vi "VFD.vi"   [LabVIEW 2018]
uses:
  CRC16/CRC16Settings.ctl
types:
  T1 = typedef "CRC16Settings.ctl" = cluster{"DataFIFO":refnum<k21>, "CalculateFIFO":refnum<k21>, "CRCFIFO":refnum<k21>}
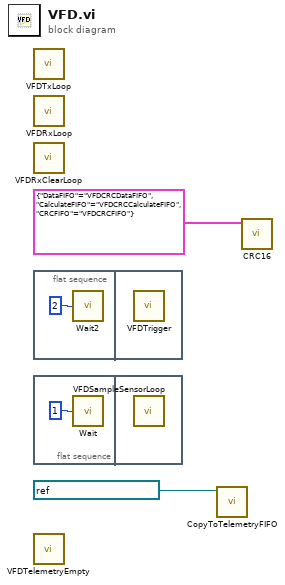
[diagram p0: block diagram]
diagram:
  n1 = call "VFDTxLoop.vi"() -> ()  [unwired: 12 in]
  n2 = call "VFDRxLoop.vi"() -> ()  [unwired: 12 in]
  n3 = call "VFDRxClearLoop.vi"() -> ()  [unwired: 12 in]
  n4 = flat-sequence {
    frame #0 {
      n5 = call "Wait2"("Count(mSec)"=u32 2) -> ()  [unwired: 1 out]
    }
    frame #1 {
      n6 = call "VFDTrigger.vi"() -> ()  [unwired: 12 in]
    }
  }
  n7 = flat-sequence {
    frame #0 {
      n8 = call "Wait"("Count(mSec)"=u32 1) -> ()  [unwired: 1 out]
    }
    frame #1 {
      n9 = call "VFDSampleSensorLoop.vi"() -> ()  [unwired: 12 in]
    }
  }
  n10 = call "VFDTelemetryEmpty.vi"() -> ()  [unwired: 12 in]
  n11 = call "CopyToTelemetryFIFO.vi"("SourceFIFO"=refnum<k21> "VFDTelemetryFIFO") -> ()  [unwired: 11 in]
  n12 = call "CRC16.vi"("CRC16Settings"=T1 {"DataFIFO"="VFDCRCDataFIFO", "CalculateFIFO"="VFDCRCCalculateFIFO", "CRCFIFO"="VFDCRCFIFO"} ("ModbusCRCSettings")) -> ()  [unwired: 11 in]
